vi "2100_Test_Rfree_Per_Throw_SP3T.vi"(0 "Semiconductor Module Context":T7, 1 "USID":T4, 2 "Publishable IDs":string[](array[string])=["R_Free", "R_Free_RF1", "R_Free_RF2", "R_Free_RF3", "R_Free_RF4"], 5 "Script_Info":T3={"Script Name"="WalkingState", "All_Scripts"=[]}, 7 "Current  Level":dbl=-0.001, 9 "Instrument_Pins":T6={"SMU_Pins"=["RF1", "RF2", "RF3", "RF4"], "HSDIO_Pins"=["CLK", "SDA"]}, 11 "Error In":errorcluster, 12 "Master_Register_Data_Array_In":T1 {"Address" format="%.0x"}, 13 "Reg_Map_and_Bit_Name":T5={"Reg_Map_Bit_Name"="", "Reg_Map"=[["Reg Addr(0x00)", "7", "6", "5", "4", "3", "2", "1", "0"], ["0", "SPARE", "RF3_SH", "RF2_SH", "RF1_SH", "SPARE", "RF3_RFC", "RF2_RFC", "RF1_RFC"], ["1", "SPARE[7:0]", "", "", "", "", "", "", ""], ["2", "VVAR_EN", "LCM_EN", "RFC_SH", "SPARE", "VARACTOR[3:0]", "", "", ""], ["3", "SW_CTRL1_VIRTUAL[7:0]", "", "", "", "", "", "", ""], ["4", "SW_CTRL1_SWAP", "SW_CTRL1_RBSHIFT[2:0]", "", "", "SW_CTRL1_VSID[3:0]", "", "", ""], ["5", "REG_00_VIRTUAL_MASK[7:0]", "", "", "", "", "", "", ""], ["6", "LOCK_STATUS[1:0]", "", "CLK_DITHER", "FUSES_BURNED", "CLK_IDAC_CAL[3:0]", "", "", ""], ["7", "SPARE[2:0]", "", "", "ODFT_TRIM[4:0]", "", "", "", ""], ["8", "SPARE[2:0]", "", "", "HV_TRIM[4:0]", "", "", "", ""], ["9", "TEST_MUX[2:0]", "", "", "SPARE[1:0]", "", "MEMS_BG_TC[1:0]", "", "MEMSCP_RCM"], ["A", "CP_BOOST_OVRD_EN", "SPARE[2:0]", "", "", "PS_OFF_TIMER[1:0]", "", "PS_ON_TIMER[1:0]", ""], ["0", "", "", "", "", "", "", "", ""], ["D", "Reserved[1:0]", "", "WD_HI_EVENT_CNT[5:0]", "", "", "", "", ""], ["E", "VERSION_ID[7:0]", "", "", "", "", "", "", ""], ["F", "Reserved", "COUNT_200_LSB[6:0]", "", "", "", "", "", ""], ["10", "CLK_DIV2_EN", "Spare", "ODFT_EN", "HV_HYST[4:0]", "", "", "", ""], ["0", "", "", "", "", "", "", "", ""], ["12", "SHORT_FUSE", "FUSE_BURN", "STROBE_EN", "VIO_OK", "RTH[1:0]", "", "FUSE_LOAD_MAN_EN", "FUSE_LOAD"], ["13", "RR_ACK_EN", "Reserved", "ACK_POSITION[1:0]", "", "SuBUS_DRIVE_STRENGTH[3:0]", "", "", ""], ["14", "TM_IO_EN", "TM_IO_SEL", "SuBUS_OVS[1:0]", "", "Reserved[3:0]", "", "", ""], ["15", "Reserved[4:0]", "", "", "", "", "SuBUS_VERSION_PRESENT", "SuBUS_VOLTAGE", "SuBUS_FLAVOR_DEF"], ["16", "PROG_STROBE1_DUR[7:0]", "", "", "", "", "", "", ""], ["17", "PROG_STROBE0_DUR[7:0]", "", "", "", "", "", "", ""], ["18", "Reserved[2:0]", "", "", "EFUSE_SINGLE_ADDR_SEL[4:0]", "", "", "", ""], ["19", "POLL_ADR[4:0]", "", "", "", "", "POLL_BC[2:0]", "", ""], ["1A", "SOFTWARE_RESET", "Reserved[6:0]", "", "", "", "", "", ""], ["1B", "Reserved[7:0]", "", "", "", "", "", "", ""], ["1C", "PWR_MODE_1", "PWR_MODE_0", "TRIGGER_MASK[2:0]", "", "", "TRIGGER[2:0]", "", ""], ["1D", "PRODUCT_ID[7:0]", "", "", "", "", "", "", ""], ["1E", "MANUFACTURER_ID_LSB[7:0]", "", "", "", "", "", "", ""], ["1F", "MANUFACTURER_ID_MSB[3:0]", "", "", "", "USID[3:0]", "", "", ""]]}) -> (6 "Master_Register_Data_Array_Out":T1 {"Address" format="%.0x"}, 15 "Error Out":errorcluster)   [LabVIEW 2013]
uses:
  Controls/USID.ctl
  <vilib>/NI_TestStand_SemiconductorModule/NI_TestStand_Semiconductor_Module.lvlibp/PinMap/General/SemiconductorModuleContext.ctl
  Controls/Master_Reg_Data_Array.ctl
  Controls/Reg_Address_Data.ctl
  <vilib>/Analysis/baseanly.llb/Mean (DBL).vi
  <vilib>/NI_TestStand_SemiconductorModule/NI_TestStand_Semiconductor_Module.lvlibp/PinMap/General/Publish/PublishDataDoubleFunctionalTest.vi
  <vilib>/NI_TestStand_SemiconductorModule/NI_TestStand_Semiconductor_Module.lvlibp
  <vilib>/Analysis/NI_AALBase.lvlib
panel:
  out "Data_Names":string[](array[string])
  out "Data_to_Log":dbl[](array[numeric])
  out "R_Measurements":dbl[][](array[numeric]) format="%#_6p"
  in  "Tab Control":enum32{"Test Info", "Instrument Settings"}(tab)
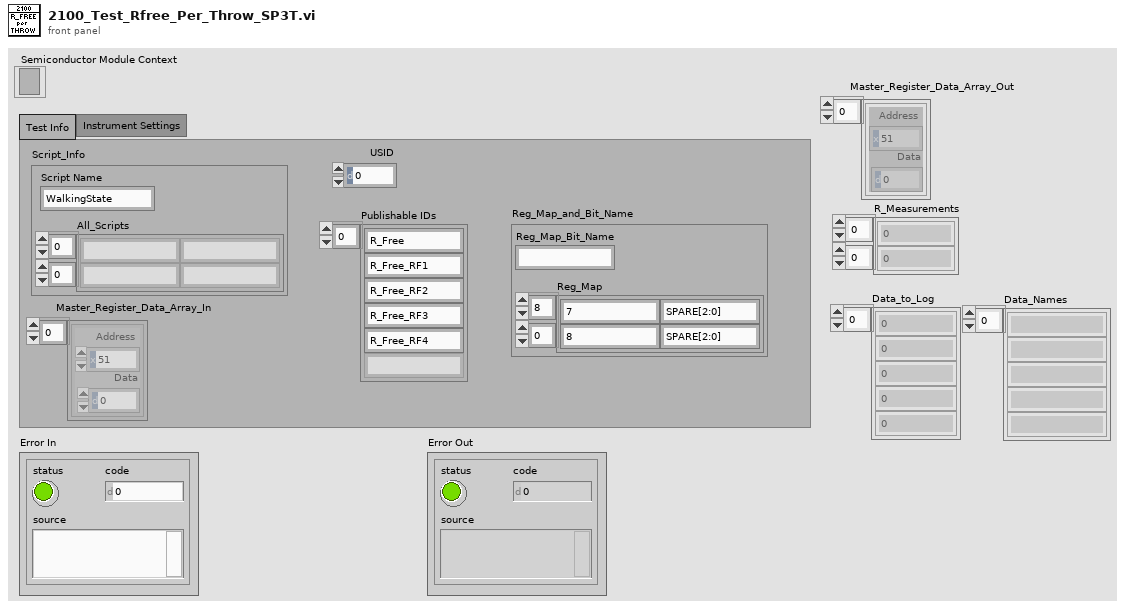
[diagram p1: front panel]
types:
  T1 = typedef "Master_Reg_Data_Array.ctl" = T2[]
  T2 = typedef "Reg_Address_Data.ctl" = cluster{"Address":u8, "Data":u8}
  T3 = cluster{"Script Name":string, "All_Scripts":string[][]}
  T4 = typedef "USID.ctl" = u8
  T5 = cluster{"Reg_Map_Bit_Name":string, "Reg_Map":string[][]}
  T6 = cluster{"SMU_Pins":string[], "HSDIO_Pins":string[]}
  T7 = typedef "NI_TestStand_Semiconductor_Module.lvlibp/SemiconductorModuleContext.ctl" = refnum<k7>
  T8 = typedef "Script Functions_Array.ctl" = enum16{"Reg_Write", "Bit_Write", "Delay", "Read", "Measure"}[]
  T9 = enum16{"Reg_Write", "Bit_Write", "Delay", "Read", "Measure"}
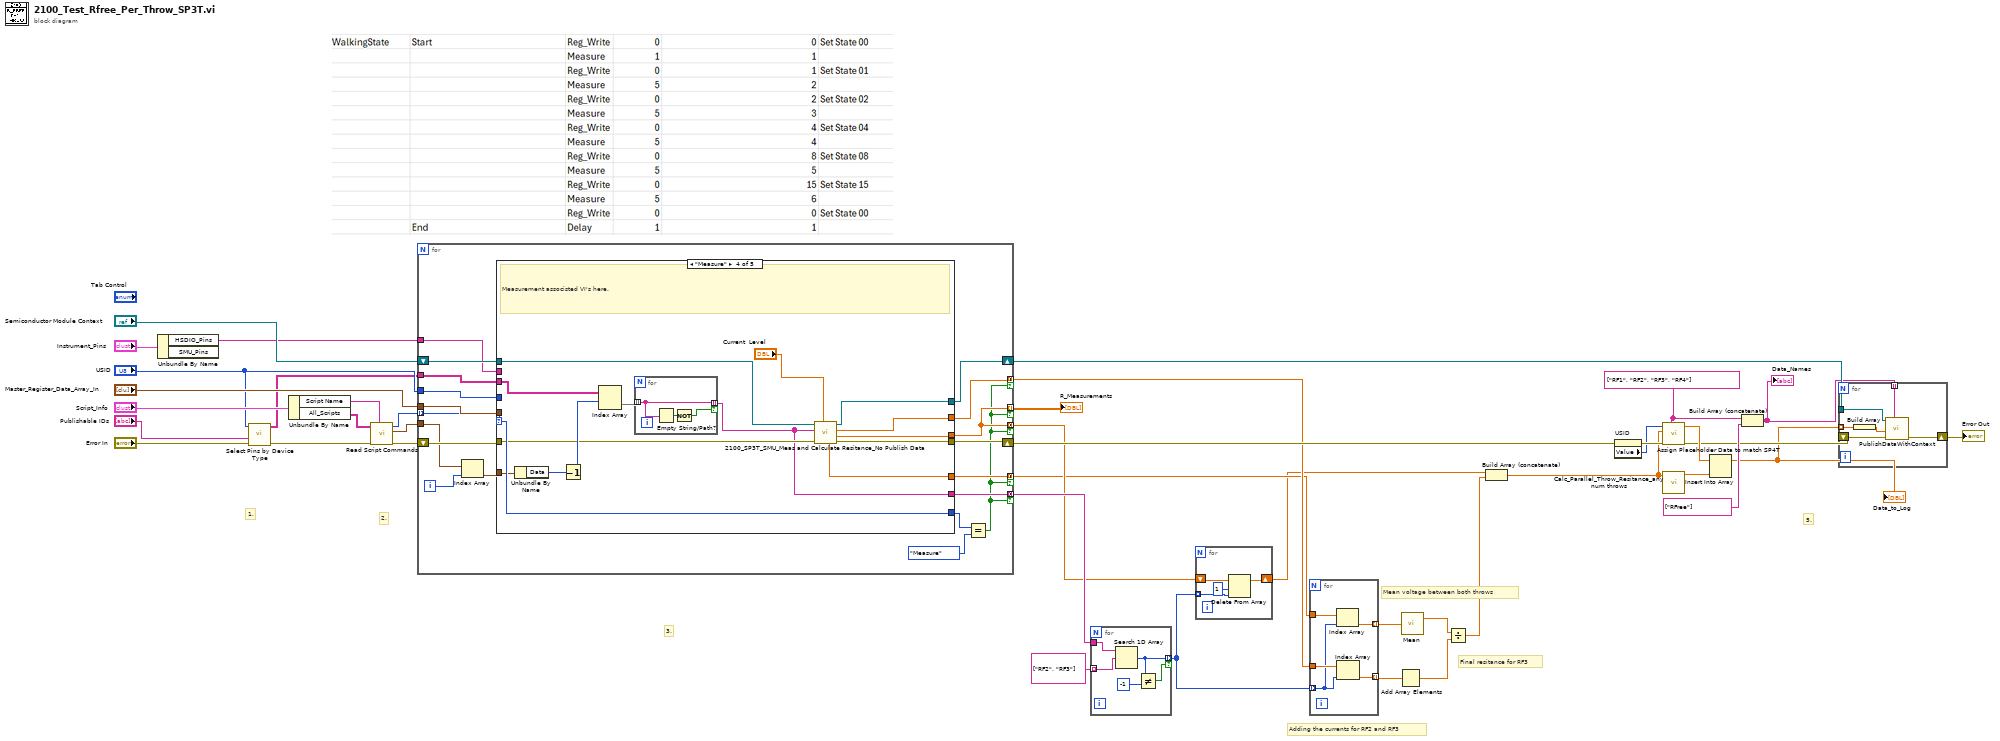
[diagram p0: block diagram]
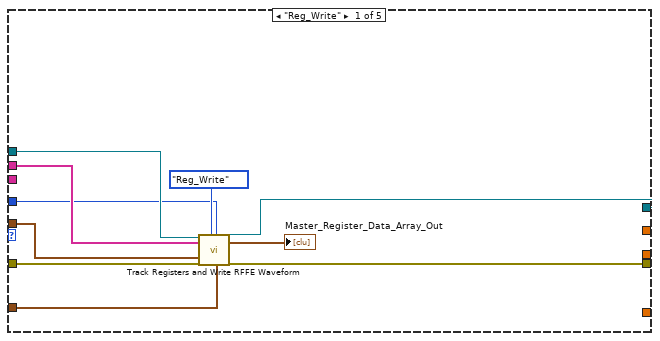
[diagram p2: hidden frame]
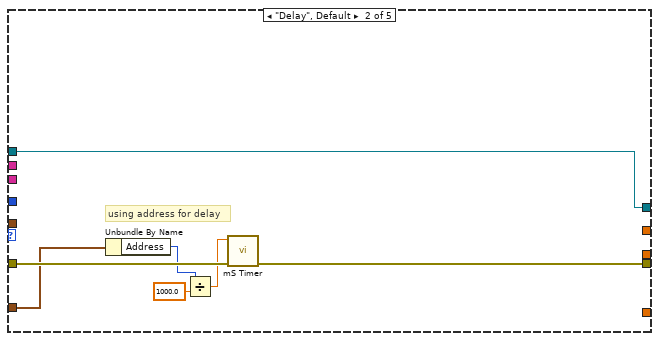
[diagram p3: hidden frame]
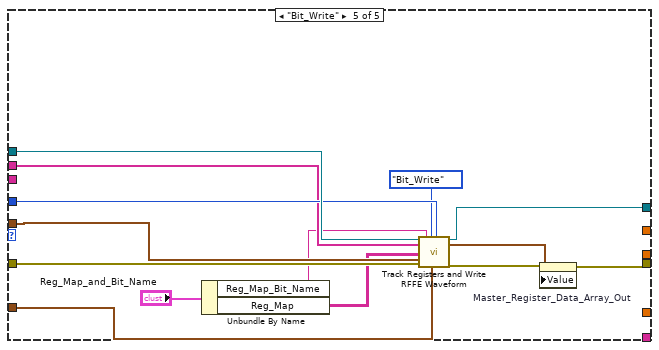
[diagram p5: hidden frame]
diagram:
  w23 = string[] ["RF1", "RF2", "RF3", "RF4"] ("SP4T_Pins")
  # "Final resitance for RF3"
  # "Mean voltage between both throws"
  # "Adding the currents for RF2 and RF3"
  # "5."
  # "3."
  # "2."
  # "1."
  n1 = Unbundle By Name("Instrument_Pins") -> ("HSDIO_Pins"=w35:string[])  [unwired: 1 out]
  n2 = call "Select Pins by Device Type.vi"("error in (no error)"="Error In", "Publishable IDs"="Publishable IDs", "USID"="USID") -> ("error out"=w28:errorcluster, "Pins to Test"=w24:string[][])  [unwired: 7 in]
  n3 = Unbundle By Name("Script_Info") -> ("Script Name"=w32:string, "All_Scripts"=w33:string[][])
  n4 = call "Read Script Commands.vi"("Test Name"=w32, "Error In"=w28, "All_Scripts"=w33) -> ("Error Out"=w39:errorcluster, "Script_Data"=w40:T2[], "Script_Functions"=w41:T8)  [unwired: 5 in, 1 out]
  n5 = for {
    tunnel: "USID" -> [w54]
    tunnel: w41 -> [w53] mode=indexing
    tunnel: w40 -> [w57]
    tunnel: w35 -> [w58]
    shift-right: [w51] -> w29
    shift-left: w39 -> [w60]
    tunnel: "Master_Register_Data_Array_In" -> [w55]
    tunnel: [w46] -> w19 mode=indexing if=w42
    shift-right: [w50] -> w30
    shift-left: "Semiconductor Module Context" -> [w59]
    tunnel: w24 -> [w47]
    tunnel: [w46] -> w11 mode=concatenating if=w42
    tunnel: [w45] -> w12 mode=concatenating if=w42
    tunnel: [w44] -> w10 mode=concatenating if=w42
    tunnel: [w43] -> w8 mode=concatenating if=w42
    i -> [w52]
    n6 = Index Array(array=w57, index=w52) -> (element=w56:T2)
    n7 = case shown="\"Measure\"" w53 {
      selector: w53 -> [_ _ _ w94 _]
      tunnel: w56 -> [w66 w76 _ w91 w98]
      tunnel: w60 -> [w70 w77 w79 w87 w111]
      tunnel: w54 -> [w63 _ _ _ w105]
      tunnel: w59 -> [w69 w71 w78 w88 w106]
      tunnel: w58 -> [w68 _ _ _ w103]
      tunnel: [w61 w75 w79 w85 w109] -> w51
      tunnel: w55 -> [w65 _ _ _ w102]
      tunnel: [w62 w71 w78 w84 w107] -> w50
      tunnel: [_ _ _ w94 _] -> w48
      tunnel: w47 -> [_ _ _ w89 _]
      tunnel: [_ _ _ w83 _] -> w46
      tunnel: [_ _ _ w86 _] -> w45
      tunnel: [_ _ _ w81 _] -> w44
      tunnel: [_ _ _ w80 _] -> w43
      frame "Reg_Write" {
        n8 = call "Track Registers and Write RFFE Waveform.vi"("Semiconductor Module Context"=w69, "Pins"=w68, "Master_Register_Data_Array_In"=w65, "Error In"=w70, "Script_Functions"=enum16{"Reg_Write", "Bit_Write"}."Reg_Write", "USID"=w63, "Reg_Address_Data"=w66) -> ("Semiconductor Module Context Out"=w62:T7, "Master_Register_Data_Array_Out"=→"Master_Register_Data_Array_Out":T1, "Error Out"=w61:errorcluster)  [unwired: 10 in]
      }
      frame "Delay", Default {
        # "using address for delay"
        n9 = Unbundle By Name(w76) -> ("Address"=w73:u8)
        n10 = Divide(x=w73, y=1000.0) -> (x/y=w72:dbl)
        n11 = call "mS Timer.vi"("Error In"=w77, "Delay(S)"=w72) -> ("Error Out"=w75:errorcluster)  [unwired: 9 in]
      }
      frame "Read" {
        # "Future Dev Code"
      }
      frame "Measure" {
        # "Measurement associsted VI's here."
        n12 = Unbundle By Name(w91) -> ("Data"=w92:u8)
        n13 = Decrement(x=w92) -> (x-1=w90:u8)
        n14 = Index Array(array=w89, index (row)=w90) -> (element=w93:string[])  [unwired: 1 in]
        n15 = for {
          tunnel: w93 -> [w97] mode=indexing
          tunnel: [w97] -> w86 mode=indexing if=w95
          n16 = Empty String/Path?(string/path=w97) -> (empty?=w96:bool)
          n17 = Not(x=w96) -> (.not. x?=w95:bool)
        }
        n18 = call "2100_SP3T_SMU_Meas and Calculate Resitance_No Publish Data.vi"("Current  Level"="Current  Level", "error in (no error)"=w87, "Pins"=w86, "Semiconductor Module Context"=w88) -> ("error Out"=w85:errorcluster, "Individual_R_Meas"=w83:dbl[], "Mean_Meas_Current"=w81:dbl[], "Semiconductor Module Context Out"=w84:T7, "Mean_Meas_Voltage"=w80:dbl[])  [unwired: 3 in]
      }
      frame "Bit_Write" {
        n19 = Unbundle By Name("Reg_Map_and_Bit_Name") -> ("Reg_Map_Bit_Name"=w100:string, "Reg_Map"=w99:string[][])
        n20 = call "Track Registers and Write RFFE Waveform.vi"("Semiconductor Module Context"=w106, "Pins"=w103, "Reg_Map"=w99, "Master_Register_Data_Array_In"=w102, "Error In"=w111, "Reg_Map_Bit_Name"=w100, "Script_Functions"=enum16{"Reg_Write", "Bit_Write"}."Bit_Write", "USID"=w105, "Reg_Address_Data"=w98) -> ("Semiconductor Module Context Out"=w107:T7, "Master_Register_Data_Array_Out"=w108:T1, "Error Out"=w110:errorcluster)  [unwired: 8 in]
        n21 = property on="Master_Register_Data_Array_Out" class="Arr (strict)"(error in=w110, "Value"=w108) -> (error out=w109:errorcluster)  [unwired: 1 in, 1 out]
      }
    }
    n22 = Equal?(x=w48, y=T9."Measure" ("Enum")) -> (x = y?=w42:bool)
  }
  "R_Measurements" <- w19
  n23 = for {
    tunnel: string[] ["RF2", "RF3"] ("SP4T_Pins") -> [w116] mode=indexing
    tunnel: [w113] -> w9 mode=indexing if=w114
    tunnel: w12 -> [w115]
    n24 = Search 1D Array(1D array=w115, element=w116) -> (index of element=w113:i32)  [unwired: 1 in]
    n25 = Not Equal?(x=w113, y=-1) -> (x != y?=w114:bool)
  }
  n26 = for {
    shift-right: [w117] -> w3
    shift-left: w11 -> [w120]
    tunnel: w9 -> [w119] mode=indexing
    n27 = Delete From Array(array=w120, length=1, index=w119) -> (array with subset deleted=w117:dbl[])  [unwired: 1 out]
  }
  n28 = for {
    tunnel: w10 -> [w125]
    tunnel: w9 -> [w122] mode=indexing
    tunnel: [w124] -> w7 mode=indexing
    tunnel: w8 -> [w123]
    tunnel: [w121] -> w6 mode=indexing
    n29 = Index Array(array=w123, index=w122) -> (element=w121:dbl)
    n30 = Index Array(array=w125, index=w122) -> (element=w124:dbl)
  }
  n31 = Add Array Elements(numeric array=w7) -> (sum=w4:dbl)
  n32 = call-poly <vilib>:"Mean.vi"("X"=w6) -> ("mean"=w5:dbl)  [unwired: 1 out]
  n33 = Divide(x=w5, y=w4) -> (x/y=w2:dbl)
  n34 = Build Array (concatenate)(w3, w2) -> (w1:dbl[])
  n35 = property on="USID" class="DigNum (strict)"(error in=w29) -> (error out=w21:errorcluster, "Value"=w20:T4)  [unwired: 1 in, 1 out]
  n36 = call "Assign Placeholder Data to match SP4T.vi"("SP4T_Pins"=w23, "error in (no error)"=w21, "Individual_R_Meas"=w1, "USID"=w20) -> ("error out"=w16:errorcluster, "Placeholder_w_Data"=w18:dbl[])  [unwired: 6 in]
  n37 = call "Calc_Parallel_Throw_Resitance_any num throws.vi"("Resitance_Per Site"=w1) -> ("Parallel_Resitance"=w17:dbl[])  [unwired: 10 in]
  n38 = Insert Into Array(array=w18, new element=w17) -> (w15:dbl[])  [unwired: 1 in]
  "Data_to_Log" <- w15
  n39 = Build Array (concatenate)(w23, string[] ["RFree"] ("element")) -> (w14:string[])
  "Data_Names" <- w14
  n40 = for {
    shift-right: [w131] -> w31
    shift-left: w16 -> [w130]
    tunnel: w30 -> [w129]
    tunnel: w15 -> [w128] mode=indexing
    tunnel: w14 -> [w126] mode=indexing
    n41 = Build Array(w128) -> (w127:dbl[])
    n42 = call-poly <vilib>:"PublishDataWithContext.vi"("Published Data Id"=w126, "error in (no error)"=w130, "Data In"=w127, "Semiconductor Module Context"=w129) -> ("error out"=w131:errorcluster)  [unwired: 6 in, 1 out]
  }
  "Error Out" <- w31
